vi "FdxCmdMonTCBSetupCvi.vi"(8 "error in":errorcluster, 9 "MonTCBSet":T1 {"ErrType" items=["FDX_TRAFFIC_SHAP_ERROR"=536870912, "FDX_SEQUENCE_NO_ERROR"=134217728, "FDX_VL_FRAME_SIZE_ERRORFDX_VL_FRAME_SIZE_ERROR"=67108864, "FDX_SHORT_FRAME_ERROR"=33554432, "FDX_LONG_FRAME_ERROR"=16777216, "FDX_NO_VALID_SFD"=8388608, "FDX_MAC_ERROR"=4194304, "FDX_IP_ERROR"=2097152, "FDX_SHORG_IFG_ERROR"=1048576, "FDX_CRC_ERROR"=524288, "FDX_TRIP_NIBBLE_ERROR"=262144, "FDX_PREAMBLE_ERROR"=131072, "FDX_RX_ERROR"=0]; "GenTrgType" items=["FDX_TRG_TCB_GEN_STD", "FDX_TRG_TCB_GEN_INV"]; "TrgType" items=["FDX_TRG_ERROR"=1, "FDX_TRG_EXTERNAL"=2, "FDX_TRG_GENERIC"=4, "FDX_TRG_VL "=8, "FDX_TRG_TIME_ABSOLUTE"=16, "FDX_TRG_TIME_DURATION"=32]}, 11 "InstrumentHandle_port":u32) -> (0 "error out":errorcluster, 3 "InstrumentHandle_port":u32)   [LabVIEW 2020, in "AIM664LV.lvlib"]
doc: "This function is used to setup one Monitor Trigger Control Block (TCB), specifying a trigger event as trigger condition. See Figure 7, which shows the dependencies and functionality of the trigger engine."
uses:
  AIM664LV.lvlib
  AFDX_LibraryAdmin/FdxGlobalDllPath.vi
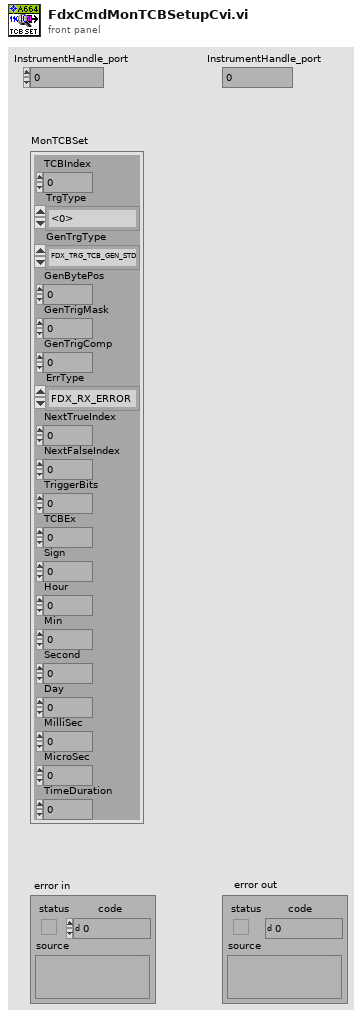
[diagram p1: front panel]
types:
  T1 = cluster{"TCBIndex":u32, "TrgType":u32, "GenTrgType":u32, "GenBytePos":u32, "GenTrigMask":u32, "GenTrigComp":u32, "ErrType":u32, "NextTrueIndex":u32, "NextFalseIndex":u32, "TriggerBits":u32, "TCBEx":u32, "Sign":i32, "Hour":u32, "Min":u32, "Second":u32, "Day":u32, "MilliSec":u32, "MicroSec":u32, "TimeDuration":u32}
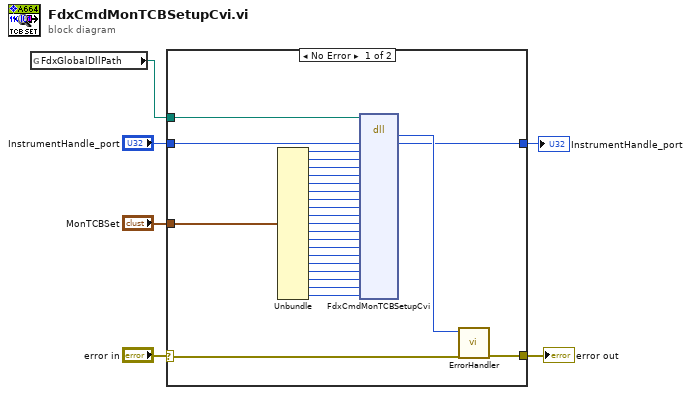
[diagram p0: block diagram]
diagram:
  n1 = global read "FdxGlobalDllPath.vi" "FdxGlobalDllPath"() -> (w4:path)
  n2 = case shown="No Error" "error in" {
    selector: "error in" -> [w31 w34]
    tunnel: [w32 w34] -> w6
    tunnel: w4 -> [w10 _]
    tunnel: "InstrumentHandle_port" -> [w9 w33]
    tunnel: [w8 w33] -> w2
    tunnel: "MonTCBSet" -> [w7 _]
    frame No Error {
      n3 = Unbundle(w7) -> ("TCBIndex"=w29:u32, "TrgType"=w28:u32, "GenTrgType"=w27:u32, "GenBytePos"=w26:u32, "GenTrigMask"=w25:u32, "GenTrigComp"=w24:u32, "ErrType"=w23:u32, "NextTrueIndex"=w22:u32, "NextFalseIndex"=w21:u32, "TriggerBits"=w20:u32, "TCBEx"=w19:u32, "Sign"=w18:i32, "Hour"=w17:u32, "Min"=w16:u32, "Second"=w15:u32, "Day"=w14:u32, "MilliSec"=w13:u32, "MicroSec"=w12:u32, "TimeDuration"=w11:u32)
      n4 = dll-call lib="aim_fdx.19.dll" fn="FdxCmdMonTCBSetupCvi"(path in=w10, "InstrumentHandle"=w9, "TCBIndex"=w29, "TrgType"=w28, "GenTrgType"=w27, "GenBytePos"=w26, "GenTrigMask"=w25, "GenTrigComp"=w24, "ErrType"=w23, "NextTrueIndex"=w22, "NextFalseIndex"=w21, "TriggerBits"=w20, "TCBEx"=w19, "Sign"=w18, "Hour"=w17, "Min"=w16, "Second"=w15, "Day"=w14, "MilliSec"=w13, "MicroSec"=w12, "TimeDuration"=w11) -> ("status"=w30:i32, "InstrumentHandle"=w8:u32)  [unwired: 21 in, 2 out]
      n5 = call "ErrorHandler.vi"("error in"=w31, "AIM Error"=w30) -> ("error out"=w32:errorcluster)  [unwired: 9 in]
    }
    frame Error {
    }
  }
  "error out" <- w6
  "InstrumentHandle_port" <- w2
